vi "XGT 연속읽기 응답 문자열 처리.vi"(10 "응답":string="\u00060ARSB010412345678\u0003") -> (1 "배열":u32[](array[numeric])=[4660, 22136] format="%.0x", 2 "에러 코드":string, 3 "데이터 개수":string="04", 5 "명령어 & 명령어 타입":string="RSB", 6 "데이터":string="12345678", 7 "국번":string="0A")   [LabVIEW 2014]
uses:
  <vilib>/regexp/Match Regular Expression.xnode
panel:
  out "숫자":u32=4
  out "Header 잘라내기":string
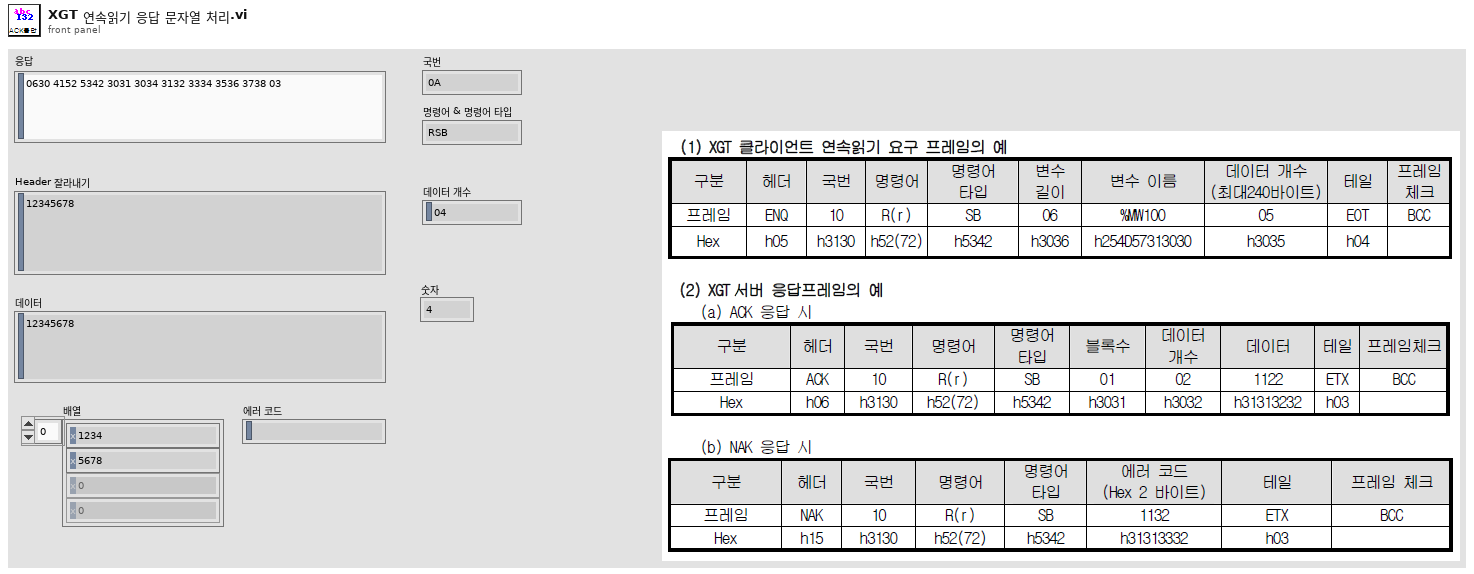
[diagram p1: front panel]
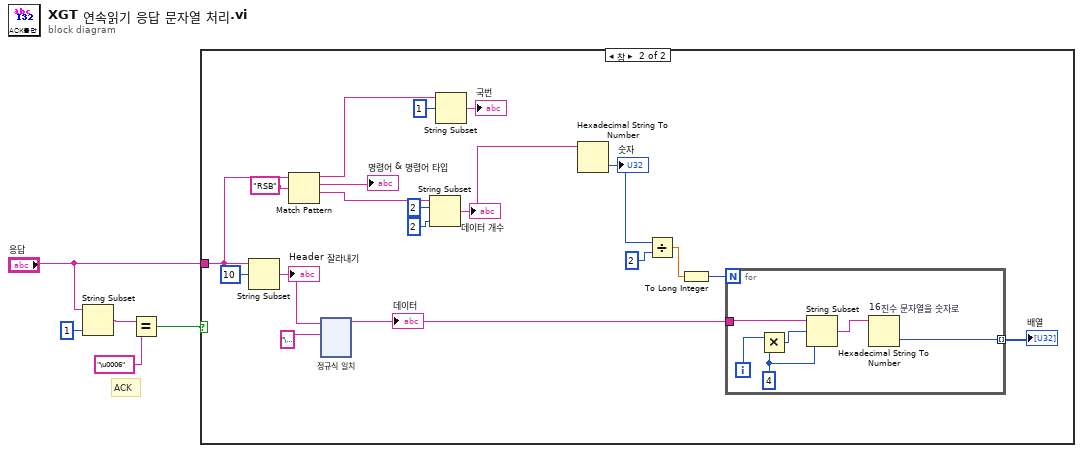
[diagram p0: block diagram]
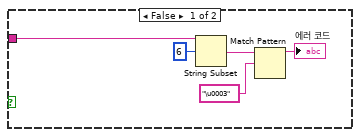
[diagram p2: hidden frame]
diagram:
  # "ACK"
  n1 = String Subset(string="응답", length (rest)=1 ("길이(나머지)")) -> (substring=w3:string)  [unwired: 1 in]
  n2 = Equal?(x=w3, y="\u0006") -> (x = y?=w1:bool)
  n3 = case shown="참" w1 {
    tunnel: "응답" -> [w10 w19]
    frame False {
      n4 = String Subset(string=w10, offset (0)=6 ("오프셋(0)")) -> (substring=w8:string)  [unwired: 1 in]
      n5 = Match Pattern(string=w8, regular expression="\u0003" ("정규식")) -> (before substring=→"에러 코드":string)  [unwired: 1 in, 3 out]
    }
    frame True {
      n6 = String Subset(string=w19, offset (0)=10 ("오프셋(0)")) -> (substring=w28:string)  [unwired: 1 in]
      "Header 잘라내기" <- w28
      n7 = Match Pattern(string=w19, regular expression="RSB" ("정규식")) -> (before substring=w22:string, match substring=→"명령어 & 명령어 타입":string, after substring=w25:string)  [unwired: 1 in, 1 out]
      n8 = xnode "정규식 일치"("입력 문자열"=w28, "정규식"="\u0003") -> ("일치 구문 앞"=w13:string)  [unwired: 4 in, 4 out]
      "데이터" <- w13
      n9 = String Subset(string=w25, offset (0)=2, length (rest)=2 ("길이(나머지)")) -> (substring=w12:string)
      "데이터 개수" <- w12
      n10 = String Subset(string=w22, offset (0)=1 ("오프셋(0)")) -> (substring=→"국번":string)  [unwired: 1 in]
      n11 = Hexadecimal String To Number(string=w12) -> (number=w15:u32)  [unwired: 2 in, 1 out]
      "숫자" <- w15
      n12 = Divide(x=w15, y=2) -> (x/y=w16:dbl)
      n13 = To Long Integer(number=w16) -> (32bit integer=w14:i32)
      n14 = for {
        N: w14 -> [_]
        tunnel: w13 -> [w35]
        tunnel: [w30] -> w11 mode=indexing
        i -> [w34]
        w32 = 4 ("y")
        n15 = Multiply(x=w34, y=w32) -> (x*y=w33:i32)
        n16 = String Subset(string=w35, offset (0)=w33, length (rest)=w32) -> (substring=w31:string)
        n17 = Hexadecimal String To Number "16진수 문자열을 숫자로"(string=w31) -> (number=w30:u32)  [unwired: 2 in, 1 out]
      }
      "배열" <- w11
    }
  }
